vi "Write JSONPayload.vi"(8 "error in (no error)":errorcluster, 10 "JSONPayload.lvclass":refnum<class "JSONPayload.lvclass">, 11 "JSONPacket in":refnum<class "JSONPacket.lvclass">) -> (0 "error out":errorcluster, 3 "JSONPacket out":refnum<class "JSONPacket.lvclass">)   [LabVIEW 2019, in "JSONPacket.lvclass"]
uses:
  JSONPacket.lvclass
  JSONPayload/JSONPayload.lvclass
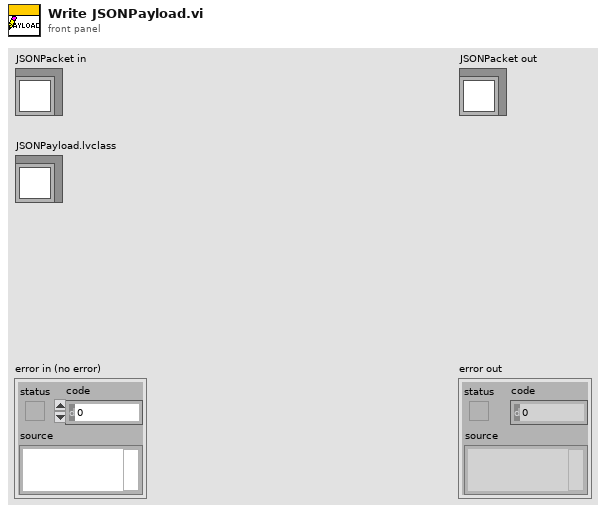
[diagram p1: front panel]
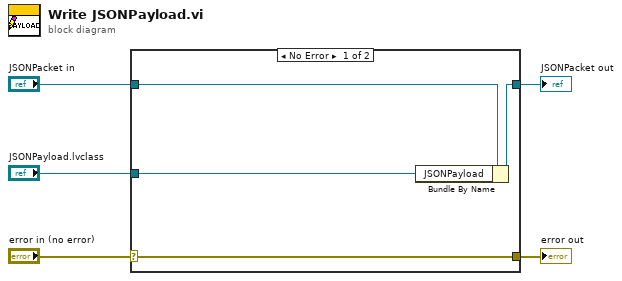
[diagram p0: block diagram]
diagram:
  n1 = case shown="No Error" "error in (no error)" {
    selector: "error in (no error)" -> [w9 w10]
    tunnel: [w9 w10] -> w4
    tunnel: [w7 w11] -> w2
    tunnel: "JSONPacket in" -> [w8 w11]
    tunnel: "JSONPayload.lvclass" -> [w6 _]
    frame No Error {
      n2 = Bundle By Name(cluster=w8, "JSONPayload"=w6) -> (w7:refnum<class "JSONPacket.lvclass">)
    }
    frame Error {
    }
  }
  "error out" <- w4
  "JSONPacket out" <- w2
